vi "niScope Configure Trigger Window.vi"(0 "instrument handle":refnum<k15>, 1 "trigger window mode":T3 items=["Entering", "Leaving"], 2 "trigger coupling":T2=1 items=["AC"=0, "DC"=1, "HF Reject"=3, "LF Reject"=4, "AC Plus HF Reject"=1001], 5 "trigger source":T1="0" caption="trigger source (Channel 0)", 7 "low level":dbl format="%.2f", 9 "high level":dbl format="%.2f", 11 "error in":errorcluster, 12 "trigger holdoff":dbl format="%.4f", 13 "trigger delay":dbl format="%.4f") -> (4 "instrument handle out":refnum<k15>, 15 "error out":errorcluster)   [LabVIEW 2020]
doc: "Configures common properties for window triggering. A window trigger occurs when a signal enters or leaves a window you specify with the <B>high level</B> or <B>low level</B> parameters."
uses:
  niScope trigger window mode.ctl
  niScope trigger coupling.ctl
  niScope trigger source.ctl
  niScope_32.dll
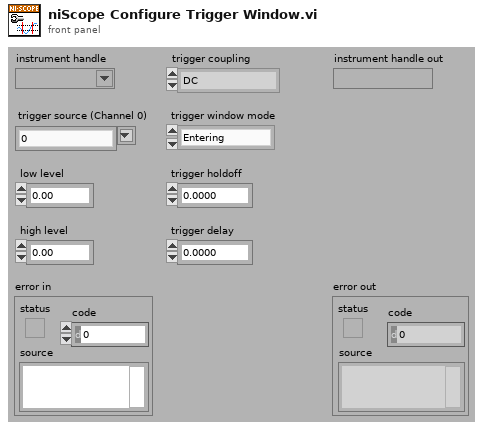
[diagram p1: front panel]
types:
  T1 = typedef "niScope trigger source.ctl" = string
  T2 = typedef "niScope trigger coupling.ctl" = u16
  T3 = typedef "niScope trigger window mode.ctl" = i32
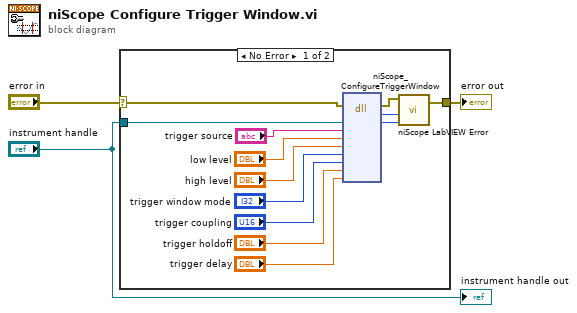
[diagram p0: block diagram]
diagram:
  n1 = case shown="No Error" "error in" {
    selector: "error in" -> [w5 w17]
    tunnel: [w13 w17] -> w3
    tunnel: "instrument handle" -> [w16 _]
    frame No Error {
      n2 = dll-call lib="niScope_*.*" fn="niScope_ConfigureTriggerWindow"(error in=w5, "instrument handle"=w16, "triggerSource"="trigger source", "lowLevel"="low level", "highLevel"="high level", "windowMode"="trigger window mode", "coupling"="trigger coupling", "holdoff"="trigger holdoff", "delay"="trigger delay") -> (error out=w4:errorcluster, "status"=w15:i32, "instrument handle"=w14:u32)  [unwired: 9 in, 1 out]
      n3 = call "niScope LabVIEW Error.vi"("instrument handle"=w14, "niScope error code (0)"=w15, "error in (no error)"=w4) -> ("error out"=w13:errorcluster)  [unwired: 2 in]
    }
    frame Error {
    }
  }
  "error out" <- w3
  "instrument handle out" <- "instrument handle"
